vi "get value from mailbox.vi"() -> ()   [LabVIEW 2012, in "Sendmail.lvrbt"]
uses:
  Sendmail.lvrbt
  <vilib>/NXT/Block Support/NXT_MessageMailbox.ctl
  <vilib>/NXT/Hardware/Plugins/Tetrix DC Motor/TetrixDCMotorAddress.ctl
  <vilib>/NXT/Dual Mode Library/BT/BlueTooth_Read_string.vi
  <vilib>/NXT/Dual Mode Library/Display/drawNumber_float.vi
  <vilib>/NXT/Dual Mode Library/Display/drawText.vi
  <vilib>/NXT/NXTIO Xnodes/NXTIONodeSubVIs/TETRIX IO Move DC Motors.vi
  <vilib>/NXT/Subs/LVHSConnector.ctl
  <vilib>/NXT/NXTIO Xnodes/AddressXNode/NXTIOAddress.xnode
  <vilib>/NXT/NXTIO Xnodes/NXTIOXNode/NXTIO.xnode
  <vilib>/NXT/LegoClasses/BrickReference/BrickReference.lvclass
panel:
  in  "String":string
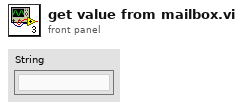
[diagram p1: front panel]
types:
  T1 = typedef "TetrixDCMotorAddress.ctl" = i16
  T2 = cluster{"TetrixDCMotor":T1, "TetrixDCMotor 2":T1}
  T3 = typedef "NXT_MessageMailbox.ctl" = u8
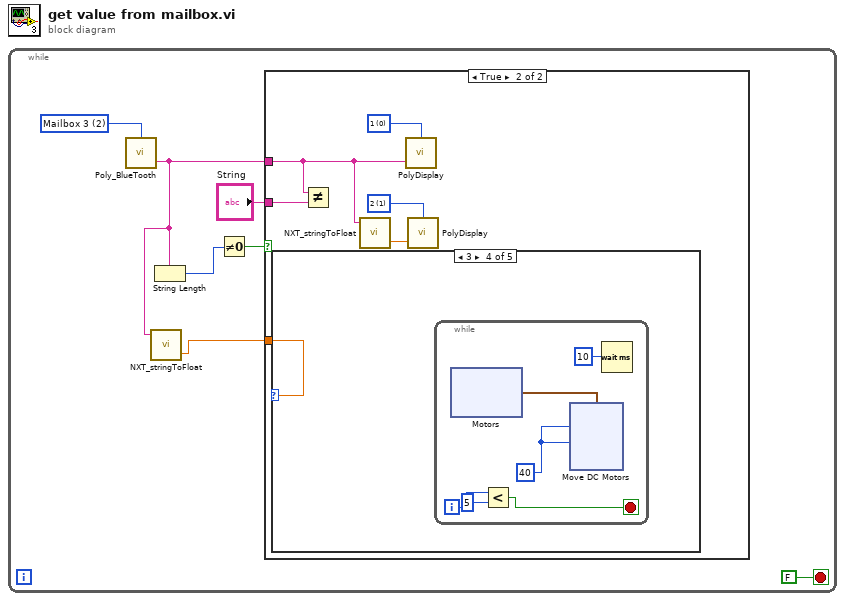
[diagram p0: block diagram]
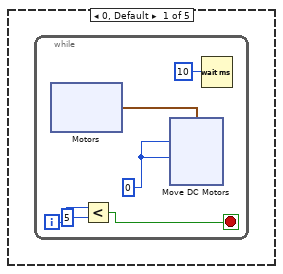
[diagram p3: hidden frame]
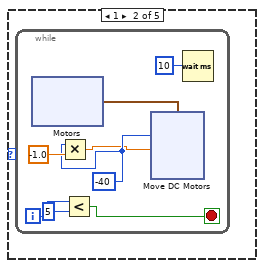
[diagram p4: hidden frame]
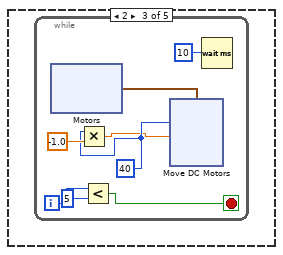
[diagram p5: hidden frame]
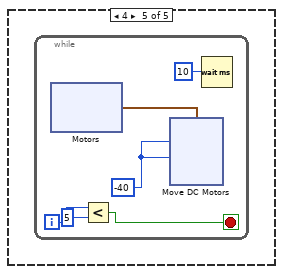
[diagram p6: hidden frame]
diagram:
  n1 = while {
    stop <- FALSE stop-if-true
    w6 = T3 2 items=["Mailbox 1", "Mailbox 2", "Mailbox 3", "Mailbox 4", "Mailbox 5", "Mailbox 6", "Mailbox 7", "Mailbox 8", "Mailbox 9", "Mailbox 10"] ("Mailbox")
    n2 = call-poly <vilib>:"Poly_BlueTooth.vi"("Mailbox"=w6) -> ("Message"=w2:string)  [unwired: 2 in, 1 out]
    n3 = call <vilib>:"NXT_stringToFloat.vi"("string"=w2) -> ("number"=w1:sgl)  [unwired: 2 in, 1 out]
    n4 = String Length(string=w2) -> (length=w3:i32)
    n5 = Not Equal To 0?(x=w3) -> (x != 0?=w7:bool)
    n6 = case shown="True" w7 {
      tunnel: w2 -> [_ w12]
      tunnel: "String" -> [_ w13]
      tunnel: w1 -> [_ w8]
      frame False {
      }
      frame True {
        w10 = i16 1 items=["1", "2", "3", "4", "5", "6", "7", "8"] ("Line")
        w11 = i16 0 items=["1", "2", "3", "4", "5", "6", "7", "8"] ("Line")
        n7 = case shown="3" w8 {
          frame 0, Default {
            n8 = while {
              i -> [w18]
              stop <- w15 stop-if-true
              w14 = 0 ("y")
              n9 = xnode "Motors"() -> ("Motor"=w19:cluster{"TetrixDCMotor":T1, "TetrixDCMotor":T1})
              n10 = Less?(x=w18, y=5) -> (x < y?=w15:bool)
              n11 = xnode "Move DC Motors"("Power/Speed 2"=w14, "Power/Speed 1"=w14, "Motors"=w19) -> ()  [unwired: 1 in, 1 out]
              n12 = Wait (ms)(milliseconds to wait=u32 10) -> ()  [unwired: 1 out]
            }
          }
          frame 1 {
            n13 = while {
              i -> [w37]
              stop <- w34 stop-if-true
              w32 = -40 ("y")
              n14 = xnode "Motors"() -> ("Motor"=w38:cluster{"TetrixDCMotor":T1, "TetrixDCMotor":T1})
              n15 = Multiply(x=w32, y=-1.0) -> (x*y=w31:dbl)
              n16 = Less?(x=w37, y=5) -> (x < y?=w34:bool)
              n17 = xnode "Move DC Motors"("Power/Speed 2"=w31, "Power/Speed 1"=w32, "Motors"=w38) -> ()  [unwired: 1 in, 1 out]
              n18 = Wait (ms)(milliseconds to wait=u32 10) -> ()  [unwired: 1 out]
            }
          }
          frame 2 {
            n19 = while {
              i -> [w56]
              stop <- w53 stop-if-true
              w51 = 40 ("y")
              n20 = xnode "Motors"() -> ("Motor"=w57:cluster{"TetrixDCMotor":T1, "TetrixDCMotor":T1})
              n21 = Multiply(x=w51, y=-1.0) -> (x*y=w50:dbl)
              n22 = Less?(x=w56, y=5) -> (x < y?=w53:bool)
              n23 = xnode "Move DC Motors"("Power/Speed 2"=w50, "Power/Speed 1"=w51, "Motors"=w57) -> ()  [unwired: 1 in, 1 out]
              n24 = Wait (ms)(milliseconds to wait=u32 10) -> ()  [unwired: 1 out]
            }
          }
          frame 3 {
            n25 = while {
              i -> [w73]
              stop <- w70 stop-if-true
              w69 = 40 ("y")
              n26 = xnode "Motors"() -> ("Motor"=w74:cluster{"TetrixDCMotor":T1, "TetrixDCMotor":T1})
              n27 = Less?(x=w73, y=5) -> (x < y?=w70:bool)
              n28 = xnode "Move DC Motors"("Power/Speed 2"=w69, "Power/Speed 1"=w69, "Motors"=w74) -> ()  [unwired: 1 in, 1 out]
              n29 = Wait (ms)(milliseconds to wait=u32 10) -> ()  [unwired: 1 out]
            }
          }
          frame 4 {
            n30 = while {
              i -> [w90]
              stop <- w87 stop-if-true
              w86 = -40 ("y")
              n31 = xnode "Motors"() -> ("Motor"=w91:cluster{"TetrixDCMotor":T1, "TetrixDCMotor":T1})
              n32 = Less?(x=w90, y=5) -> (x < y?=w87:bool)
              n33 = xnode "Move DC Motors"("Power/Speed 2"=w86, "Power/Speed 1"=w86, "Motors"=w91) -> ()  [unwired: 1 in, 1 out]
              n34 = Wait (ms)(milliseconds to wait=u32 10) -> ()  [unwired: 1 out]
            }
          }
        }
        n35 = Not Equal?(x=w12, y=w13) -> ()  [unwired: 1 out]
        n36 = call <vilib>:"NXT_stringToFloat.vi"("string"=w12) -> ("number"=w9:sgl)  [unwired: 2 in, 1 out]
        n37 = call-poly <vilib>:"PolyDisplay.vi"("Text"=w12, "Line"=w11) -> ()  [unwired: 2 in, 1 out]
        n38 = call-poly <vilib>:"PolyDisplay.vi"("number"=w9, "Line"=w10) -> ()  [unwired: 2 in, 1 out]
      }
    }
  }
